vi "SVL Limit Testing (cluster of x0, dx, array) (scalar limits).vi"(8 "error in (no error)":errorcluster, 9 "lower limit":dbl=-inf format="%.2f", 10 "upper limit":dbl=inf format="%.2f", 11 "signal in":cluster{"x0":dbl, "dx":dbl, "array":dbl[]} {"array" format="%.2f"; "dx" format="%.2p"; "x0" format="%.2p"}) -> (0 "error out":errorcluster, 1 "output values":cluster{"f0":dbl, "df":dbl, "spectrum":dbl[]}[](graph), 2 "test results":bool[](array[boolean]), 3 "test passed?":bool)   [LabVIEW 2017, in "SoundVib_LimitTest.lvlib"]
doc: "Performs limit testing on waveforms, spectra, XY data, identified peaks, or scalar measurements. You can specify an upper and lower boundary of the envelope to define a pass range. This VI uses the defined pass range to test the input signal. VI outputs apply only to the current input signal. You can wire output values to a graph to view the limits, signal, and failures. Wire data to the<B> signal in</B> input to determine the polymorphic instance to use or manually select the instance."
uses:
  <vilib>/addons/Sound and Vibration/svt_Limit Test/SoundVib_LimitTest.lvlib
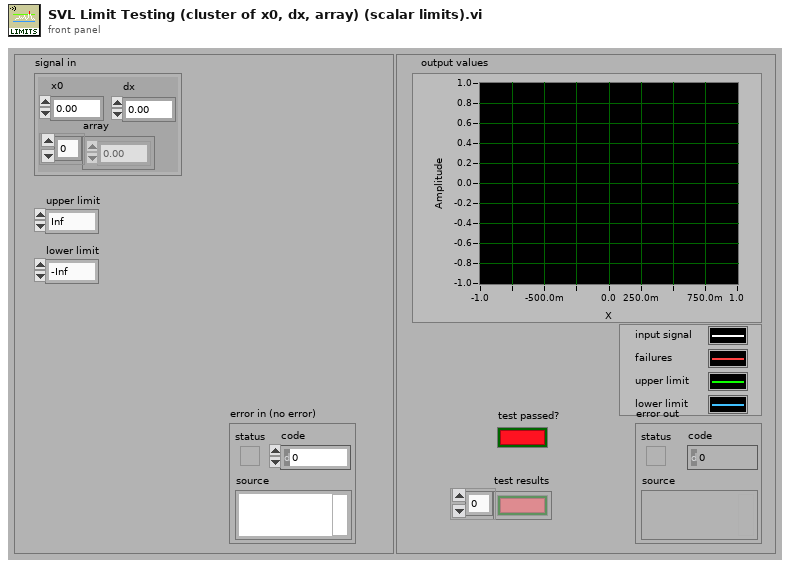
[diagram p1: front panel]
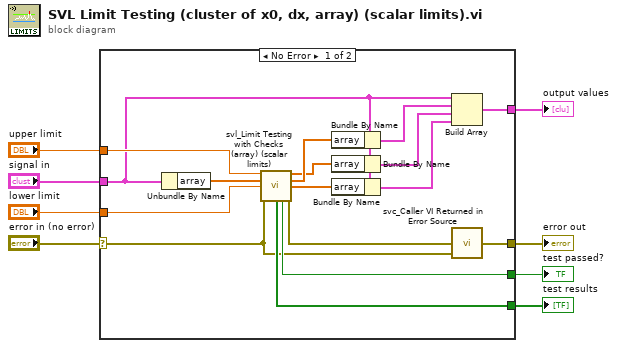
[diagram p0: block diagram]
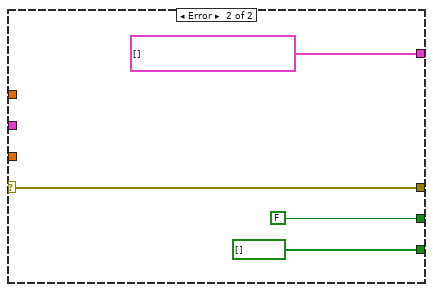
[diagram p2: hidden frame]
diagram:
  n1 = case shown="No Error" "error in (no error)" {
    selector: "error in (no error)" -> [w9 w28]
    tunnel: [w23 w28] -> w7
    tunnel: [w15 cluster{"f0":dbl, "df":dbl, "spectrum":dbl[]}[] []] -> w6
    tunnel: [w18 bool[] [] ("Array Constant")] -> w5
    tunnel: [w19 FALSE] -> w4
    tunnel: "upper limit" -> [w22 _]
    tunnel: "signal in" -> [w14 _]
    tunnel: "lower limit" -> [w21 _]
    frame No Error {
      n2 = Unbundle By Name(w14) -> ("array"=w24:dbl[])
      n3 = call <vilib>:"svl_Limit Testing with Checks (array) (scalar limits).vi"("upper limit"=w22, "input array"=w24, "lower limit"=w21, "error in (no error)"=w9) -> ("upper limit array"=w10:dbl[], "failure array"=w11:dbl[], "lower limit array"=w16:dbl[], "test results"=w18:bool[], "test passed"=w19:bool, "error out"=w20:errorcluster)  [unwired: 6 in]
      n4 = Bundle By Name(cluster=w14, "array"=w11) -> (w12:cluster{"x0":dbl, "dx":dbl, "array":dbl[]})
      n5 = Bundle By Name(cluster=w14, "array"=w10) -> (w13:cluster{"x0":dbl, "dx":dbl, "array":dbl[]})
      n6 = Bundle By Name(cluster=w14, "array"=w16) -> (w17:cluster{"x0":dbl, "dx":dbl, "array":dbl[]})
      n7 = Build Array(w14, w12, w13, w17) -> (w15:cluster{"x0":dbl, "dx":dbl, "array":dbl[]}[])
      n8 = call <vilib>:"svc_Caller VI Returned in Error Source.vi"("warning input to caller"=w9, "error in (no error)"=w20) -> ("error out"=w23:errorcluster)  [unwired: 3 in]
    }
    frame Error {
    }
  }
  "error out" <- w7
  "output values" <- w6
  "test passed?" <- w4
  "test results" <- w5
